vi "RisingEdge.vi"(11 "Input":bool) -> (3 "Rising?":bool)   [LabVIEW 2015]
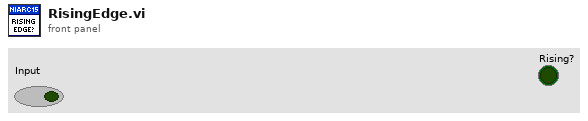
[diagram p1: front panel]
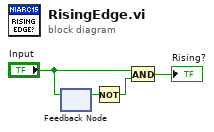
[diagram p0: block diagram]
diagram:
  n1 = feedback #1() -> (w4:bool)  [unwired: 1 in]
  n2 = feedback-in #1("Input") -> ()
  n3 = Not(x=w4) -> (.not. x?=w3:bool)
  n4 = And(x="Input", y=w3) -> (x .and. y?=→"Rising?":bool)
